vi "change tag select name.vi"(8 "error in":errorcluster, 9 "new name":string, 10 "old name":string, 11 "tag select module configuration in":refnum<class "Table Test configuration.lvclass">) -> (0 "error out":errorcluster, 1 "new channels":refnum<class "TBM channel.lvclass">[](array[class]), 2 "old channels":refnum<class "TBM channel.lvclass">[](array[class]), 3 "tag select module configuration out":refnum<class "Table Test configuration.lvclass">)   [LabVIEW 2013, in "Table Test configuration.lvclass"]
uses:
  Table Test configuration.lvclass
  <vilib>/NI/Tag Bus Module Framework/channel/TBM channel.lvclass
  Table Test configuration.lvclass/Table Test configuration.ctl
  <vilib>/NI/Tag Bus/tag/tag descriptor.lvclass/tag descriptor.ctl
  <vilib>/NI/Tag Bus/tag/tag descriptor.lvclass
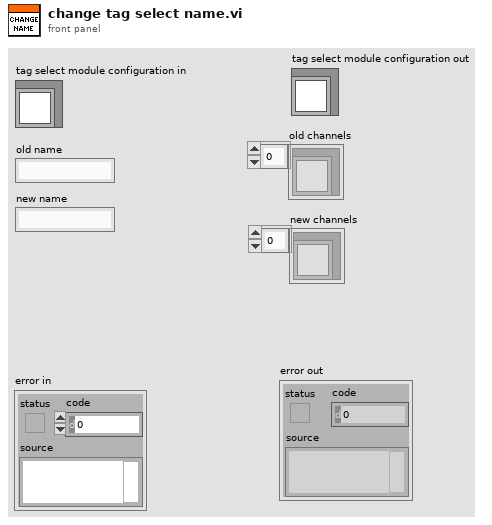
[diagram p1: front panel]
types:
  T1 = typedef "Table Test configuration.lvclass/tag select configuration.ctl" = cluster{"tag select name":string, "data type":T2, "output":refnum<class "TBM channel.lvclass">, "select":refnum<class "TBM channel.lvclass">, "input channels":refnum<class "TBM channel.lvclass">[]}
  T2 = typedef "tag bus.lvlib/tag descriptor.lvclass/Data Type.ctl" = enum16{"Double", "Single", "I64", "I32", "I16", "I8", "U64", "U32", "U16", "U8", "Boolean", "String", "Array of Double", "Array of Single", "Array of I64", "Array of I32", "Array of I16", "Array of I8", "Array of U64", "Array of U32", "Array of U16", "Array of U8", "Array of Boolean", "Array of String"}
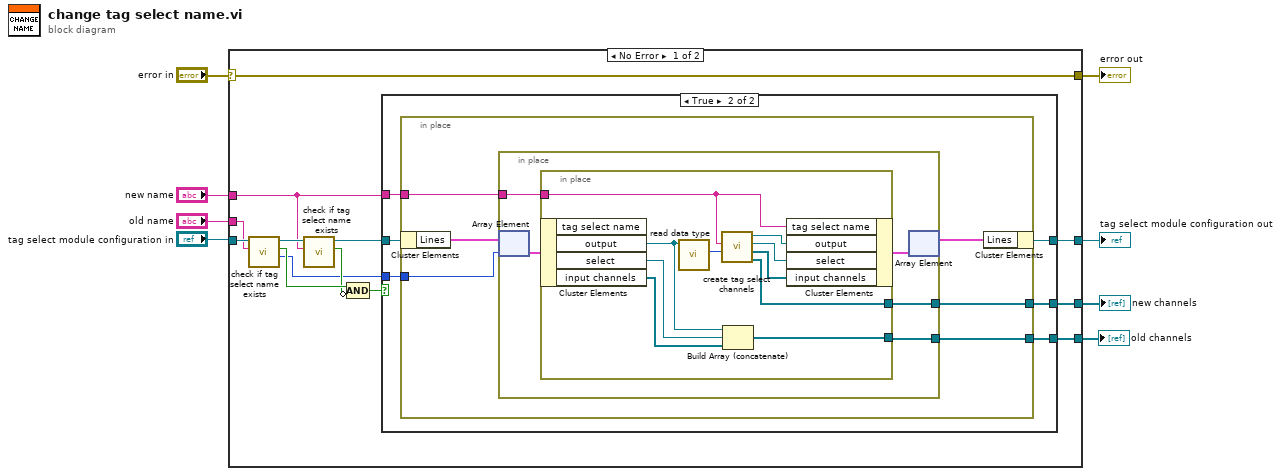
[diagram p0: block diagram]
diagram:
  n1 = case shown="No Error" "error in" {
    selector: "error in" -> [w21 w51]
    tunnel: [w21 w51] -> w7
    tunnel: [w18 w50] -> w6
    tunnel: "tag select module configuration in" -> [w20 w50]
    tunnel: "old name" -> [w19 _]
    tunnel: "new name" -> [w11 _]
    tunnel: [w10 _] -> w3
    tunnel: [w9 _] -> w2
    frame No Error {
      n2 = call "check if tag select name exists.vi"("name to locate"=w19, "tag select module configuration in"=w20) -> ("index"=w12:i32, "found?"=w15:bool, "tag select module configuration out"=w17:refnum<class "Table Test configuration.lvclass">)  [unwired: 6 in, 1 out]
      n3 = call "check if tag select name exists.vi"("name to locate"=w11, "tag select module configuration in"=w17) -> ("found?"=w14:bool, "tag select module configuration out"=w16:refnum<class "Table Test configuration.lvclass">)  [unwired: 6 in, 2 out]
      n4 = Compound Arithmetic op=AND(w15, invert w14) -> (w13:bool)
      n5 = case shown="True" w13 {
        tunnel: w16 -> [w22 w28]
        tunnel: [w22 w27] -> w18
        tunnel: w12 -> [_ w26]
        tunnel: w11 -> [_ w25]
        tunnel: [_ w24] -> w10
        tunnel: [_ w23] -> w9
        frame False {
        }
        frame True {
          n6 = in-place {
            in-place-border: w26 -> [w32]
            in-place-border: w25 -> [w31]
            in-place-border: [w30] -> w24
            in-place-border: [w29] -> w23
            n7 = in-place-cluster #1(w28) -> ("Lines"=w34:T1[])
            n8 = in-place {
              in-place-border: w31 -> [w38]
              in-place-border: [w36] -> w30
              in-place-border: [w35] -> w29
              n9 = in-place-array #2(w34, w32) -> (w39:T1)
              n10 = in-place {
                in-place-border: w38 -> [w45]
                in-place-border: [w44] -> w36
                in-place-border: [w40] -> w35
                n11 = in-place-cluster #3(w39) -> ("output"=w43:refnum<class "TBM channel.lvclass">, "select"=w42:refnum<class "TBM channel.lvclass">, "input channels"=w41:refnum<class "TBM channel.lvclass">[])  [unwired: 1 out]
                n12 = call <vilib>:"read data type.vi"("system tag in"=w43) -> ("data type"=w49:T2)  [unwired: 8 in, 2 out]
                n13 = call "create tag select channels.vi"("data type"=w49, "tag select name"=w45) -> ("created channels"=w44:refnum<class "TBM channel.lvclass">[], "inputs"=w46:refnum<class "TBM channel.lvclass">[], "select"=w47:refnum<class "TBM channel.lvclass">, "output"=w48:refnum<class "TBM channel.lvclass">)  [unwired: 6 in]
                n14 = Build Array (concatenate)(w43, w42, w41) -> (w40:refnum<class "TBM channel.lvclass">[])
                n15 = in-place-cluster #3("tag select name"=w45, "output"=w48, "select"=w47, "input channels"=w46) -> (w37:T1)
              }
              n16 = in-place-array #2(w37) -> (w33:T1[])  [unwired: 1 out]
            }
            n17 = in-place-cluster #1("Lines"=w33) -> (w27:refnum<class "Table Test configuration.lvclass">)
          }
        }
      }
    }
    frame Error {
    }
  }
  "error out" <- w7
  "tag select module configuration out" <- w6
  "new channels" <- w3
  "old channels" <- w2
